vi "Step Move X.vi"(2 "Error In":errorcluster, 3 "Direction":bool=TRUE, 4 "No. of X Steps":string="0", 5 "Reference In":refnum<class "_Controller.lvclass">) -> (0 "Error Out":errorcluster, 1 "Reference Out":refnum<class "_Controller.lvclass">)   [LabVIEW 2020]
doc: "Moves the XYZ scanning machine in the X-direction. \n\nArgs:\n\nReference In: Incoming communication (reference) between LabView and the scanning rig controller\nError In: Checks for any errors with the incoming communication (reference)\nNo. of X Steps: Number of steps the motor needs to move\nDirection: Boolean to control the direction the motor moves in \n\nReturns: \n\nReference Out: Output communnication (reference) between LabView and controller\nError Out: Checks for any error with output communication (reference)"
uses:
  <instrlib>/Arcus Ethernet Driver 1.0.0/ArcusEthernetComm/classes/Controller/_Controller.lvclass
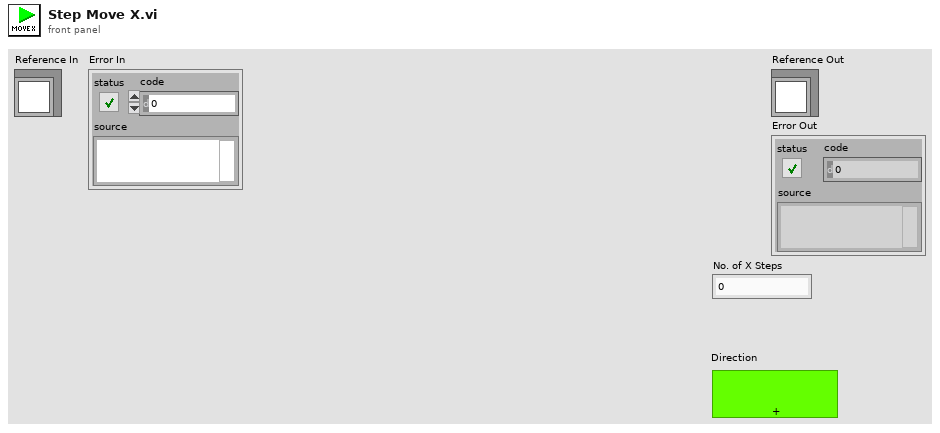
[diagram p1: front panel]
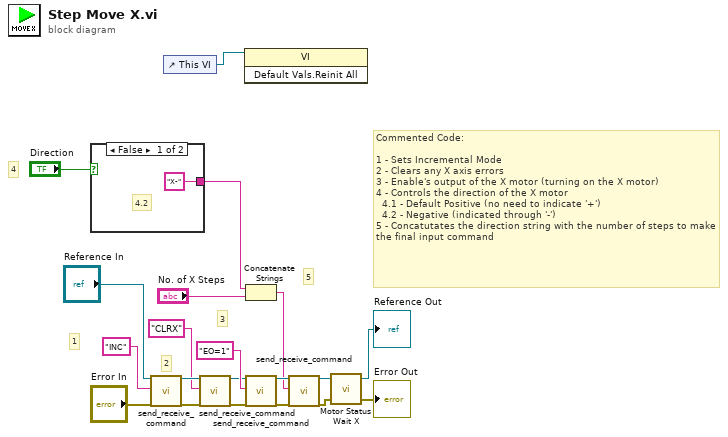
[diagram p0: block diagram]
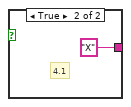
[diagram p2: hidden frame]
diagram:
  # "Commented Code:\n\n1 - Sets Incremental Mode \n2 - Clears any X axis errors\n3 - Enable's output of the X motor (turning on the X motor)\n4 - Controls the direction of the X motor\n  4.1 - Default Positive (no need to indicate '+')\n  4.2 - Negative (indicated through '-') \n5 - Concatutates the direction string with the number of steps to make the final input command"
  # "5"
  # "4"
  # "2"
  # "3"
  # "1"
  n1 = case shown="False" "Direction" {
    tunnel: ["X-" "X"] -> w9
    frame False {
      # "4.2"
    }
    frame True {
      # "4.1"
    }
  }
  n2 = call <instrlib>:"send_receive_command.vi"("reference (in)"="Reference In", "ASCII Command (in)"="INC", "error in (no error)"="Error In") -> ("reference (out)"=w19:refnum<class "_Controller.lvclass">, "error out"=w20:errorcluster)  [unwired: 12 in, 3 out]
  n3 = control-ref of="This VI"() -> (w2:refnum<vi>)
  n4 = call <instrlib>:"send_receive_command.vi"("reference (in)"=w19, "ASCII Command (in)"="CLRX", "error in (no error)"=w20) -> ("reference (out)"=w14:refnum<class "_Controller.lvclass">, "error out"=w13:errorcluster)  [unwired: 12 in, 3 out]
  n5 = invoke class="VI" method="Default Vals.Reinit All"(reference=w2) -> ()  [unwired: 2 in, 3 out]
  n6 = Concatenate Strings(w9, "No. of X Steps") -> (w8:string)
  n7 = call <instrlib>:"send_receive_command.vi"("reference (in)"=w14, "ASCII Command (in)"="EO=1", "error in (no error)"=w13) -> ("reference (out)"=w16:refnum<class "_Controller.lvclass">, "error out"=w15:errorcluster)  [unwired: 12 in, 3 out]
  n8 = call <instrlib>:"send_receive_command.vi"("reference (in)"=w16, "ASCII Command (in)"=w8, "error in (no error)"=w15) -> ("reference (out)"=w3:refnum<class "_Controller.lvclass">, "error out"=w1:errorcluster)  [unwired: 12 in, 3 out]
  n9 = call "Motor Status Wait X.vi"("Error In"=w1, "Reference In"=w3) -> ("Error Out"=→"Error Out":errorcluster, "Reference Out"=→"Reference Out":refnum<class "_Controller.lvclass">)  [unwired: 2 in]
